vi "Launch Nested Actors.vi"(8 "error in (no error)":errorcluster, 11 "BuildServer in":refnum<class "BuildServer.lvclass">) -> (0 "error out":errorcluster, 3 "BuildServer out":refnum<class "BuildServer.lvclass">)   [LabVIEW 2017, in "BuildServer.lvlib" / "BuildServer.lvclass"]
uses:
  BuildServer.lvclass
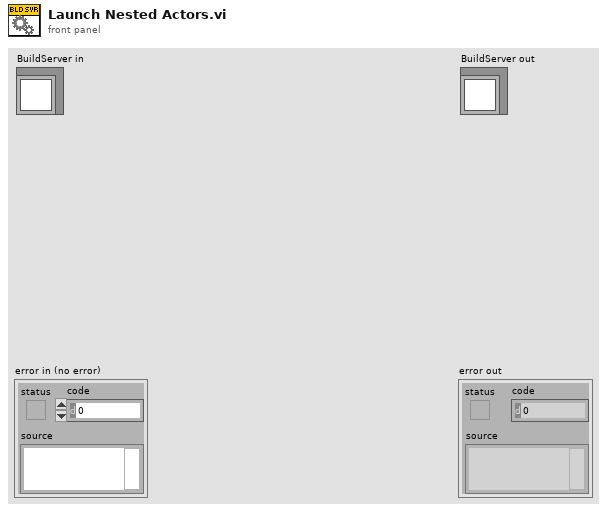
[diagram p1: front panel]
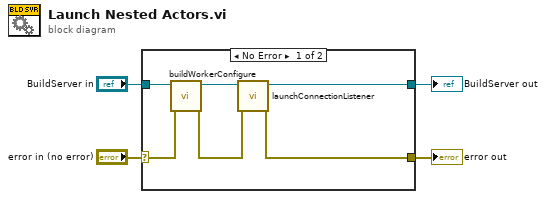
[diagram p0: block diagram]
diagram:
  n1 = case shown="No Error" "error in (no error)" {
    selector: "error in (no error)" -> [w6 w12]
    tunnel: [w5 w12] -> w3
    tunnel: [w8 w11] -> w1
    tunnel: "BuildServer in" -> [w10 w11]
    frame No Error {
      n2 = call "buildWorkerConfigure.vi"("error in (no error)"=w6, "BuildServer in"=w10) -> ("error out"=w7:errorcluster, "BuildServer out"=w9:refnum<class "BuildServer.lvclass">)  [unwired: 8 in]
      n3 = call "launchConnectionListener.vi"("error in (no error)"=w7, "BuildServer in"=w9) -> ("error out"=w5:errorcluster, "BuildServer out"=w8:refnum<class "BuildServer.lvclass">)  [unwired: 8 in]
    }
    frame Error {
    }
  }
  "error out" <- w3
  "BuildServer out" <- w1
